vi "Launch Module.vi"(11 "Error in":errorcluster caption="Error in (no error)") -> (15 "Error out":errorcluster)   [LabVIEW 2019, in "GP Module.lvlib"]
doc: "<Developer>\nGPower\n21/9 2019"
uses:
  Actors/Module/GP Module.lvlib
  <vilib>/GPower/Logger/Library/Logger Class/Logger/Severity Level.ctl
  <vilib>/GPower/Logger - MCL/Library/MCL Logger Class/MCL Logger.lvclass
  C:/Program Files (x86)/National Instruments/LabVIEW 2019/vi.lib/GPower/Logger/Library/Logger Class/Logger.lvclass
  Actors/Module/Module Class/Module.lvclass
  C:/Program Files (x86)/National Instruments/LabVIEW 2019/vi.lib/GPower/Actor/Library/Actor Class/Actor.lvclass
  <vilib>/GPower/Actor/Library/Final Message Class/Accessors/Decode Final Message (No Cast).vi
  <vilib>/GPower/Actor/Library/Actor Class/Actor.lvclass
  <vilib>/GPower/Actor/Library/Actor Interface Class/Actor Interface.lvclass
  <vilib>/GPower/Message/Library/Message Class/Message.lvclass
  <vilib>/GPower/Actor/Library/Final Message Class/Final Message.lvclass
  <vilib>/GPower/Logger/Library/Logger Class/Logger.lvclass
panel:
  in  "Multicolumn Listbox":i32(listbox)
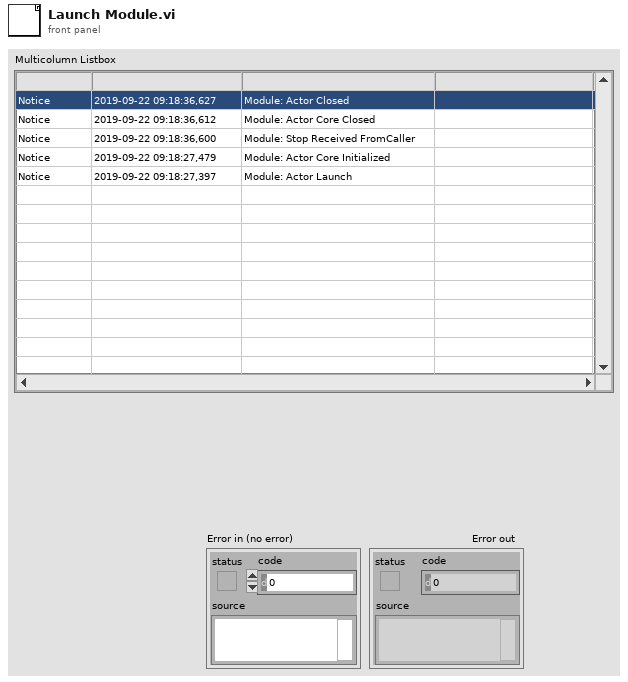
[diagram p1: front panel]
types:
  T1 = typedef "GP Logger.lvlib/Logger.lvclass/Severity Level.ctl" = enum16{"Emergency", "Alert", "Critical", "Error", "Warning", "Notice", "Info", "Debug"}
  T2 = typedef "GP Actor.lvlib/Actor Interface.lvclass/Registered Actor Events.ctl" = cluster{"Actor Messages":refnum<event-registration>, "Actor Stopped":refnum<event-registration>, "Actor Stop":refnum<event-registration>}
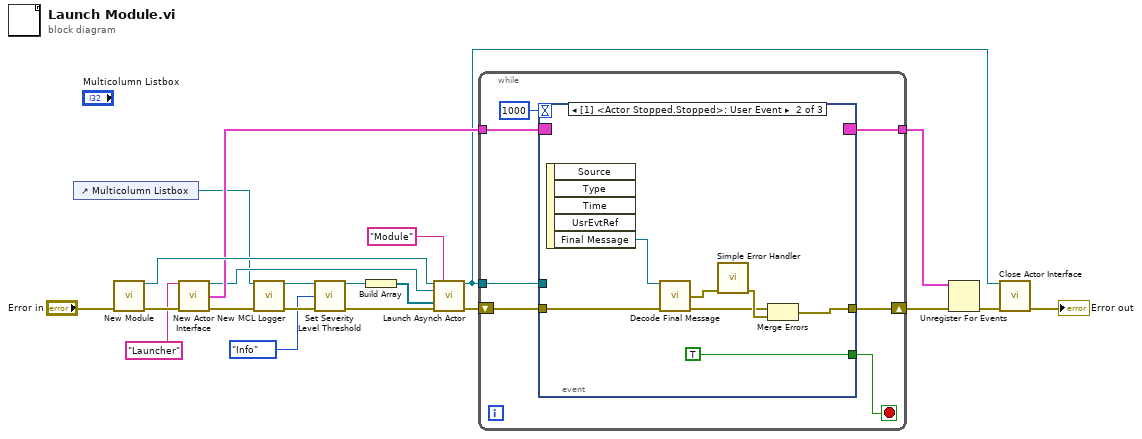
[diagram p0: block diagram]
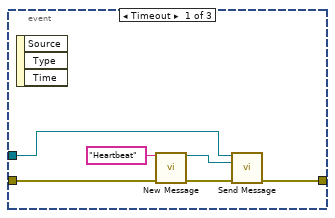
[diagram p2: hidden frame]
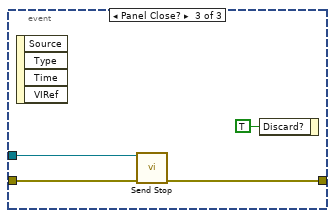
[diagram p3: hidden frame]
diagram:
  n1 = control-ref of="Multicolumn Listbox"() -> (w15:refnum<vi>)
  n2 = call "New Module.vi"("Error in"="Error in") -> ("New Module"=w20:refnum<class "Module.lvclass">, "Error out"=w19:errorcluster)  [unwired: 13 in]
  n3 = call <vilib>:"New Actor Interface.vi"("My Name"="Launcher", "Error in"=w19) -> ("New Actor Interface"=w16:refnum<class "Actor Interface.lvclass">, "Registered Actor Events"=w17:T2, "Error out"=w14:errorcluster)  [unwired: 11 in]
  n4 = call <vilib>:"New MCL Logger.vi"("Multicolumn Listbox"=w15, "Error in"=w14) -> ("MCL Logger"=w5:refnum<class "MCL Logger.lvclass">, "Error out"=w3:errorcluster)  [unwired: 12 in]
  n5 = call <vilib>:"Set Severity Level Threshold.vi"("Logger in"=w5, "Severity Level Threshold"=Severity_Level."Info", "Error in"=w3) -> ("Logger out"=w4:refnum<class "MCL Logger.lvclass">, "Error out"=w2:errorcluster)  [unwired: 11 in]
  n6 = Build Array(w4) -> (w13:refnum<class "MCL Logger.lvclass">[])
  n7 = call <vilib>:"Launch Asynch Actor.vi"("Actor"=w20, "Actor Name"="Module", "Caller Interface"=w16, "Loggers"=w13, "Error in"=w2) -> ("Actor Interface"=w6:refnum<class "Actor Interface.lvclass">, "Error out"=w12:errorcluster)  [unwired: 9 in]
  n8 = while {
    tunnel: w17 -> [w28]
    shift-right: [w26] -> w10
    shift-left: w12 -> [w27]
    tunnel: w6 -> [w25]
    tunnel: [w22] -> w9
    stop <- w23 stop-if-true
    n9 = event shown="[1] <Actor Stopped.Stopped>: User Event" {
      selector: w28 -> [_ _ _]
      dyn-events: [_ _ _] -> w22
      timeout: 1000 -> [_ _ _]
      tunnel: w27 -> [w32 w41 w45]
      tunnel: [w34 w36 w44] -> w26
      tunnel: w25 -> [w33 _ w43]
      tunnel: [_ TRUE _] -> w23
      event Timeout {
        n10 = event-data() -> ()  [unwired: 1 in, 3 out]
        n11 = call <vilib>:"New Message.vi"("Name"="Heartbeat", "Error in"=w32) -> ("New Message"=w30:refnum<class "Message.lvclass">, "Error out"=w31:errorcluster)  [unwired: 12 in]
        n12 = call <vilib>:"Send Message.vi"("Receiver"=w33, "Message"=w30, "error in (no error)"=w31) -> ("error out"=w34:errorcluster)  [unwired: 12 in]
      }
      event User Event {
        n13 = event-data() -> ("Final Message"=w40:refnum<class "Final Message.lvclass">)  [unwired: 1 in, 4 out]
        n14 = call-poly <vilib>:"Decode Final Message.vi"("Final Message in"=w40, "Error in"=w41) -> ("Actor Final Error"=w39:errorcluster, "Error out"=w37:errorcluster)  [unwired: 9 in, 3 out]
        n15 = call <vilib>:"Simple Error Handler.vi"("error in (no error)"=w39) -> ("error out"=w38:errorcluster)  [unwired: 4 in, 4 out]
        n16 = Merge Errors(w37, w38) -> (w36:errorcluster)
      }
      event Panel Close? {
        n17 = event-data() -> ()  [unwired: 1 in, 4 out]
        n18 = call <vilib>:"Send Stop.vi"("Receiver"=w43, "Error in"=w45) -> ("Error out"=w44:errorcluster)  [unwired: 13 in]
        n19 = event-data("Discard?"=TRUE) -> ()  [unwired: 1 in, 1 out]
      }
    }
  }
  n20 = Unregister For Events(event registration refnum=w9, error in=w10) -> (error out=w8:errorcluster)
  n21 = call <vilib>:"Close Actor Interface.vi"("Actor Interface"=w6, "Error in"=w8) -> ("Error out"=→"Error out":errorcluster)  [unwired: 13 in]
